vi "connect.vi"(0 "Module ID":i32=-1, 5 "ip":string, 7 "S_port":dbl, 9 "R_port":dbl, 11 "error in":errorcluster, 12 "timeout":dbl) -> (15 "error out":errorcluster)   [LabVIEW 2024, in "cameraV1.lvlib"]
doc: "_____\nCreated using DQMH Framework: Event Scripter 7.1.0.1503."
uses:
  cameraV1.lvlib
  connect Argument--cluster.ctl
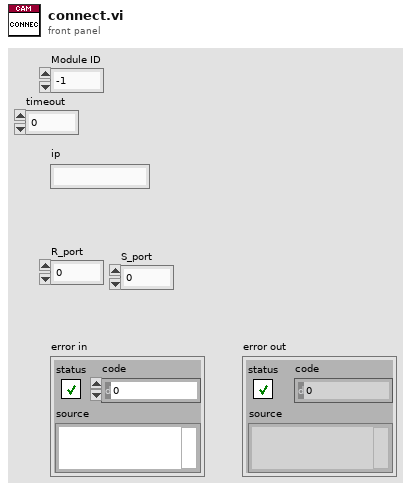
[diagram p1: front panel]
types:
  T1 = typedef "cameraV1.lvlib/connect Argument--cluster.ctl" = cluster{"Module ID":i32, "ip":string, "R_port":dbl, "S_port":dbl, "timeout":dbl}
  T2 = typedef "cameraV1.lvlib/Request Events--cluster.ctl" = cluster{"Stop Module":refnum<user-event>, "Show Panel":refnum<user-event>, "Hide Panel":refnum<user-event>, "Show Diagram":refnum<user-event>, "Get Module Execution Status":refnum<user-event>, "connect":refnum<user-event>, "Send_Command":refnum<user-event>, "Cam Image Response":refnum<user-event>}
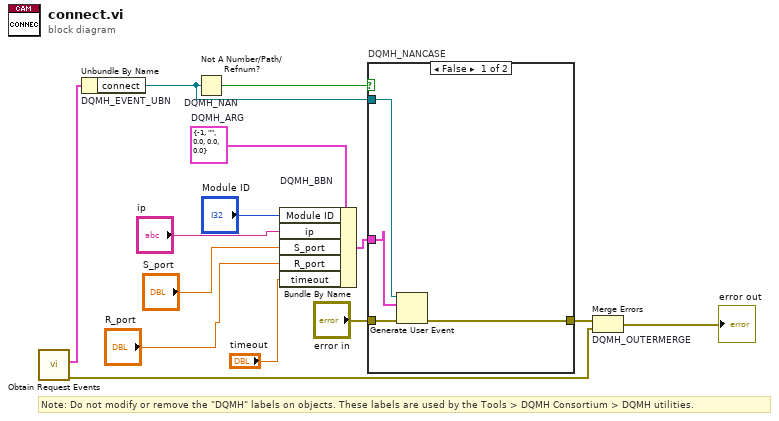
[diagram p0: block diagram]
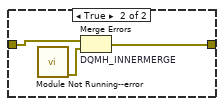
[diagram p2: hidden frame]
diagram:
  w9 = T1 {"Module ID"=-1, "ip"="", "R_port"=0.0, "S_port"=0.0, "timeout"=0.0}  # DQMH_ARG
  # "Note: Do not modify or remove the \"DQMH\" labels on objects. These labels are used by the Tools > DQMH Consortium > DQMH utilities."
  n1 = call "Obtain Request Events.vi"() -> ("error out"=w6:errorcluster, "cameraV1 Request Events"=w5:T2)  [unwired: 10 in]
  n2 = Unbundle By Name "DQMH_EVENT_UBN"(w5) -> ("connect"=w11:refnum<user-event>)
  n3 = Not A Number/Path/Refnum? "DQMH_NAN"(number/path/refnum=w11) -> (NaN/Path/Refnum?=w12:bool)
  n4 = Bundle By Name "DQMH_BBN"(cluster=w9, "Module ID"="Module ID", "ip"="ip", "S_port"="S_port", "R_port"="R_port", "timeout"="timeout") -> (w2:T1)
  n5 = case "DQMH_NANCASE" shown="False" w12 {
    tunnel: "error in" -> [w18 w21]
    tunnel: [w17 w20] -> w10
    tunnel: w11 -> [w16 _]
    tunnel: w2 -> [w15 _]
    frame False {
      n6 = Generate User Event(user event=w16, event data cluster=w15, error in=w18) -> (error out=w17:errorcluster)  [unwired: 1 in, 1 out]
    }
    frame True {
      n7 = call "Module Not Running--error.vi"() -> ("error out"=w19:errorcluster)  [unwired: 11 in]
      n8 = Merge Errors "DQMH_INNERMERGE"(w21, w19) -> (w20:errorcluster)
    }
  }
  n9 = Merge Errors "DQMH_OUTERMERGE"(w10, w6) -> (→"error out":errorcluster)
